vi "GetChannelSettings.vi"(8 "error in (no error)":errorcluster, 11 "TektronixDPO in":refnum<class "TektronixDPO.lvclass">) -> (0 "error out":errorcluster, 3 "TektronixDPO out":refnum<class "TektronixDPO.lvclass">)   [LabVIEW 2013, in "TektronixDPO.lvclass"]
uses:
  TektronixDPO.lvclass
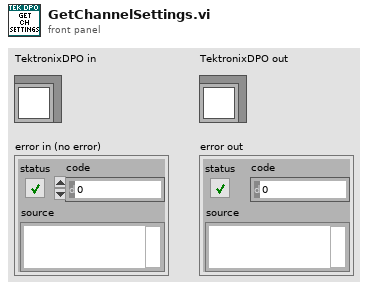
[diagram p1: front panel]
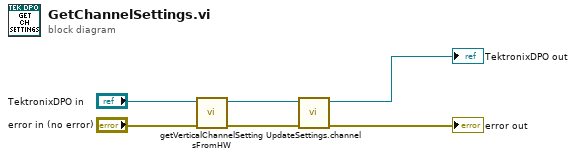
[diagram p0: block diagram]
diagram:
  n1 = call "getVerticalChannelSettingsFromHW.vi"("error in (no error)"="error in (no error)", "TektronixDPO in"="TektronixDPO in") -> ("error out"=w2:errorcluster, "TektronixDPO out"=w1:refnum<class "TektronixDPO.lvclass">)  [unwired: 8 in]
  n2 = call "UpdateSettings.channel.vi"("error in (no error)"=w2, "TektronixDPO in"=w1) -> ("error out"=→"error out":errorcluster, "TektronixDPO out"=→"TektronixDPO out":refnum<class "TektronixDPO.lvclass">)  [unwired: 8 in]
